vi "XY Graph to Igor Graph.vi"(8 "error in (no error)":errorcluster, 9 "Filename":string="testname", 10 "Path":path=path "C:/temp", 11 "XY Graph Reference":refnum<vi>) -> (0 "error out":errorcluster, 2 "file":path=path "C:/Users/voodoo.SEAGATE/Desktop/datatest/datatest.000019.itx")   [LabVIEW 2016, in "LV to ITX.lvclass"]
uses:
  LV to ITX.lvclass
  <userlib>/LevyLab/Graph Utilities/graph_utilities.lvclass/graph_utilities.ctl
  <userlib>/LevyLab/Graph Utilities/graph_utilities.lvclass
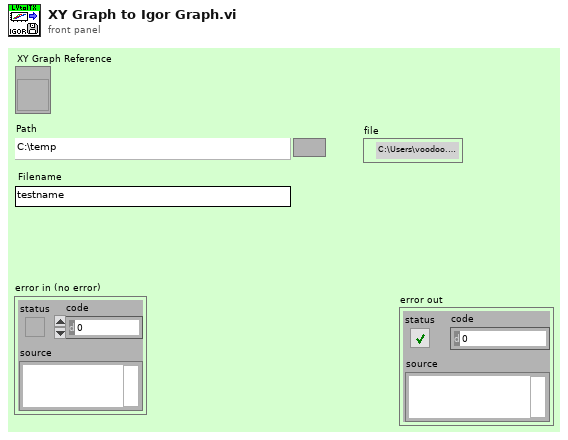
[diagram p1: front panel]
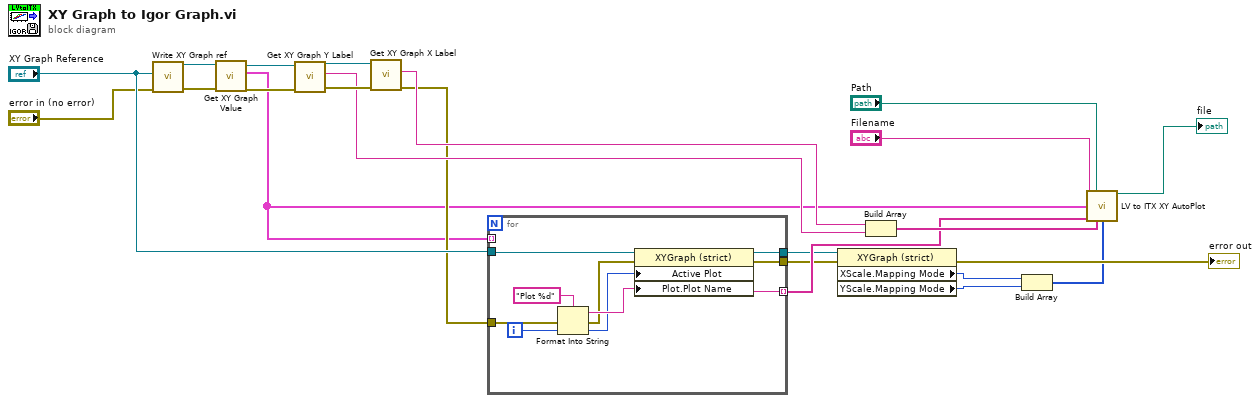
[diagram p0: block diagram]
diagram:
  n1 = call <userlib>:"Write XY Graph ref.vi"("error in (no error)"="error in (no error)", "XY Graph"="XY Graph Reference") -> ("error out"=w17:errorcluster, "graph_utilities out"=w18:refnum<class "graph_utilities.lvclass">)  [unwired: 8 in]
  n2 = call <userlib>:"Get XY Graph Value.vi"("error in (no error)"=w17, "graph_utilities in"=w18) -> ("error out"=w15:errorcluster, "Value"=w2:cluster{"X":dbl[], "Y":dbl[]}[], "graph_utilities out"=w16:refnum<class "graph_utilities.lvclass">)  [unwired: 7 in]
  n3 = call <userlib>:"Get XY Graph Y Label.vi"("error in (no error)"=w15, "graph_utilities in"=w16) -> ("error out"=w13:errorcluster, "Y Label"=w11:string, "graph_utilities out"=w14:refnum<class "graph_utilities.lvclass">)  [unwired: 7 in]
  n4 = call <userlib>:"Get XY Graph X Label.vi"("error in (no error)"=w13, "graph_utilities in"=w14) -> ("error out"=w6:errorcluster, "X Label"=w12:string)  [unwired: 7 in, 1 out]
  n5 = for {
    tunnel: [w28] -> w9 mode=indexing
    tunnel: "XY Graph Reference" -> [w31]
    tunnel: [w30] -> w8
    tunnel: w2 -> [_] mode=indexing
    tunnel: w6 -> [w26]
    tunnel: [w24] -> w5
    i -> [w27]
    n6 = Format Into String(format string="Plot %d", error in=w26, w27) -> (resulting string=w28:string, error out=w25:errorcluster)  [unwired: 1 in]
    n7 = property on="Property Node" class="XYGraph (strict)"(reference=w31, error in=w25, "Active Plot"=w27, "Plot.Plot Name"=w28) -> (reference out=w30:refnum<vi>, error out=w24:errorcluster)
  }
  n8 = property on="Property Node" class="XYGraph (strict)"(reference=w8, error in=w5) -> (error out=→"error out":errorcluster, "XScale.Mapping Mode"=w21:u8, "YScale.Mapping Mode"=w20:u8)  [unwired: 1 out]
  n9 = Build Array(w12, w11) -> (w22:string[])
  n10 = Build Array(w21, w20) -> (w3:u8[])
  n11 = call "LV to ITX XY AutoPlot.vi"("filename"="Filename", "path"="Path", "XY Array"=w2, "wavenames (.Vx, etc)"=w9, "X,Y Labels"=w22, "X,Y Log"=w3) -> ("file"=→"file":path)  [unwired: 9 in]
